vi "TTA_EXA_ACPRMode.vi"(0 "VISA resource In":refnum<visa-resource-name>, 5 "Frequency (MHz)":dbl, 7 "State File":path, 11 "error in":errorcluster) -> (4 "VISA resource Out":refnum<visa-resource-name>, 15 "error out":errorcluster)   [LabVIEW 2016]
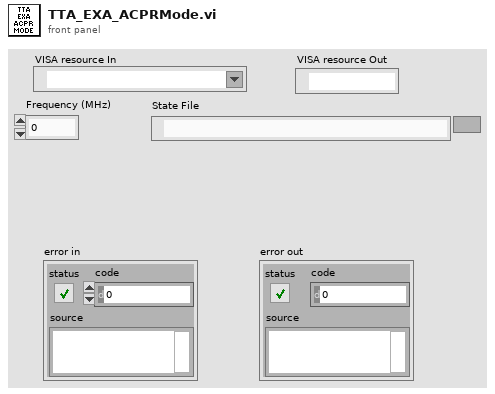
[diagram p1: front panel]
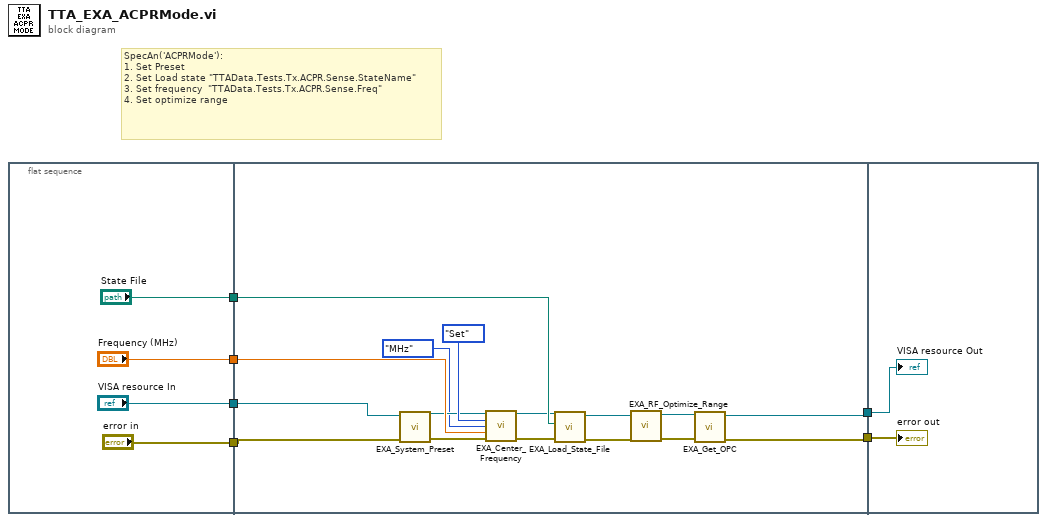
[diagram p0: block diagram]
diagram:
  # "SpecAn('ACPRMode'):\n1. Set Preset\n2. Set Load state \"TTAData.Tests.Tx.ACPR.Sense.StateName\"\n3. Set frequency  \"TTAData.Tests.Tx.ACPR.Sense.Freq\"\n4. Set optimize range"
  n1 = flat-sequence {
    tunnel: ["error in"] -> w6
    tunnel: ["VISA resource In"] -> w5
    tunnel: ["Frequency (MHz)"] -> w4
    tunnel: ["State File"] -> w1
    tunnel: w6 -> [w20]
    tunnel: w5 -> [w19]
    tunnel: w4 -> [w25]
    tunnel: [w12] -> w3
    tunnel: [w11] -> w2
    tunnel: w1 -> [w18]
    tunnel: w3 -> [w28]
    tunnel: w2 -> [w27]
    frame #0 {
    }
    frame #1 {
      n2 = call "EXA_System_Preset.vi"("error in"=w20, "VISA resource name"=w19) -> ("error out"=w26:errorcluster, "VISA resource name"=w23:refnum<visa-resource-name>)  [unwired: 8 in]
      n3 = call "EXA_Center_Frequency.vi"("VISA resource name"=w23, "Mode"=enum16{"Set", "Get"}."Set", "Units"=enum16{"Hz", "kHz", "MHz", "GHz"}."MHz", "Frequency"=w25, "error in"=w26) -> ("VISA resource name"=w17:refnum<visa-resource-name>, "error out"=w16:errorcluster)  [unwired: 8 in, 1 out]
      n4 = call "EXA_Load_State_File.vi"("error in"=w16, "Path"=w18, "VISA resource name"=w17) -> ("error out"=w21:errorcluster, "VISA resource name"=w15:refnum<visa-resource-name>)  [unwired: 7 in]
      n5 = call "EXA_RF_Optimize_Range.vi"("error in"=w21, "VISA resource name"=w15) -> ("error out"=w14:errorcluster, "VISA resource name"=w13:refnum<visa-resource-name>)  [unwired: 8 in]
      n6 = call "EXA_Get_OPC.vi"("error in"=w14, "VISA resource name"=w13) -> ("error out"=w11:errorcluster, "VISA resource name"=w12:refnum<visa-resource-name>)  [unwired: 7 in, 1 out]
    }
    frame #2 {
      "VISA resource Out" <- w28
      "error out" <- w27
    }
  }
